vi "Build Update Str.vi"(5 "sel":string, 7 "update":string, 8 "error in (no error)":errorcluster, 10 "Col":string, 11 "code":string) -> (0 "error out":errorcluster, 2 "Update":string, 3 "Sel":string)   [LabVIEW 2014]
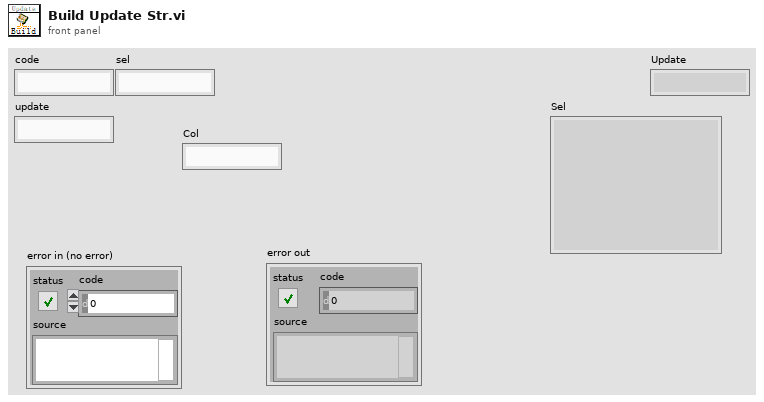
[diagram p1: front panel]
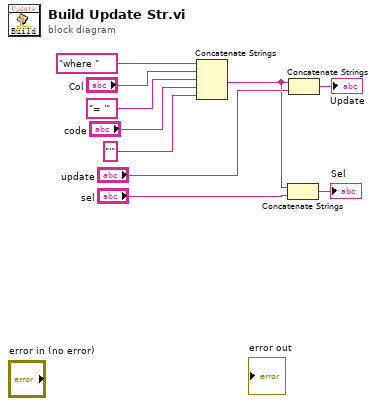
[diagram p0: block diagram]
diagram:
  n1 = Concatenate Strings("where ", "Col", "= '", "code", "'" ("Col 2")) -> (w4:string)
  n2 = Concatenate Strings(w4, "sel") -> (→"Sel":string)
  n3 = Concatenate Strings(w4, "update") -> (→"Update":string)
